vi "CASH.vi"(8 "error in (no error)":errorcluster caption="entrée d'erreur (pas d'erreur)", 11 "Portfolio en entrée":refnum<class "Portfolio.lvclass"> caption="DNL_LabVIEW Object in") -> (0 "error out":errorcluster caption="sortie d'erreur", 2 "CASH":dbl, 3 "Portfolio en sortie":refnum<class "Portfolio.lvclass"> caption="DNL_LabVIEW Object out")   [LabVIEW 2012, in "Portfolio.lvclass"]
uses:
  Portfolio.lvclass
  Portfolio.lvclass/Portfolio.ctl
  Operations/Operations.lvclass
  Exchanges/Exchanges.lvclass
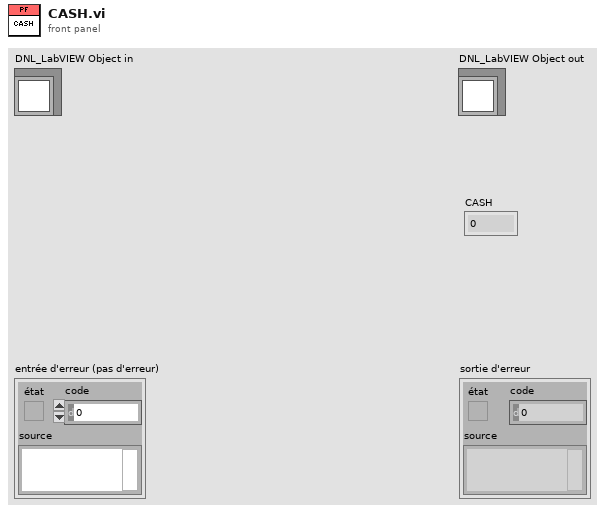
[diagram p1: front panel]
types:
  T1 = typedef "Operation Parameters.ctl" = cluster{"Date":timestamp, "Operation Type":T2, "Amount":dbl, "Comment":string, "Currency":T3}
  T2 = typedef "Operation Type Enum.ctl" = enum16{"Coupons", "Dépot", "Retrait", "Intérêts", "Taxe"}
  T3 = typedef "Currencies.ctl" = enum16{"Euro", "Dollar", "Yen", "RIM", "CHF"}
  T4 = typedef "Exchange Parameters.ctl" = cluster{"Date":timestamp, "Exchange Type":T5, "ISIN":string, "Label":string, "Price":dbl, "Qty":dbl, "Currency":T3, "Tax":dbl, "Comment":string}
  T5 = typedef "Exchange.lvclass/Exchange Type Enum.ctl" = enum16{"ACHAT", "VENTE"}
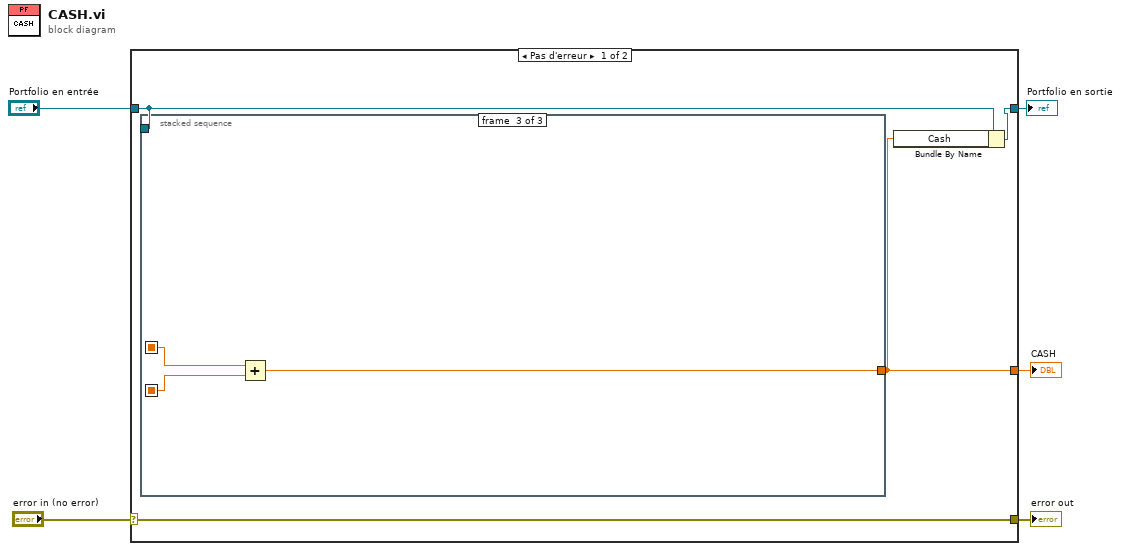
[diagram p0: block diagram]
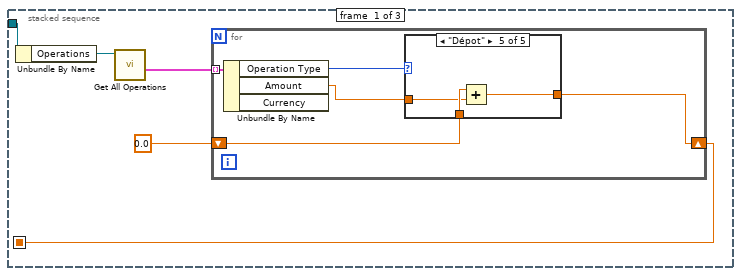
[diagram p2: hidden frame]
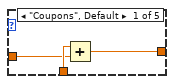
[diagram p3: hidden frame]
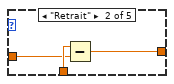
[diagram p4: hidden frame]
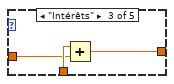
[diagram p5: hidden frame]
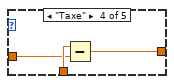
[diagram p6: hidden frame]
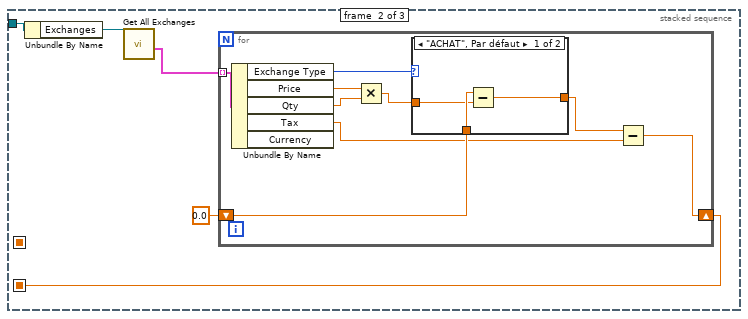
[diagram p7: hidden frame]
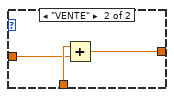
[diagram p8: hidden frame]
diagram:
  n1 = case shown="Pas d'erreur" "error in (no error)" {
    selector: "error in (no error)" -> [w9 w59]
    tunnel: [w9 w59] -> w4
    tunnel: [w7 w58] -> w2
    tunnel: "Portfolio en entrée" -> [w8 w58]
    tunnel: [w6 _] -> w1
    frame No Error {
      n2 = stacked-sequence {
        seq-local: [w10 _ _] -> [_ _ w57]
        seq-local: [_ w35 _] -> [_ _ w56]
        tunnel: w8 -> [w14 w39 _]
        tunnel: [_ _ w55] -> w6
        frame #0 {
          n3 = Unbundle By Name(w14) -> ("Operations"=w13:refnum<class "Operations.lvclass">)
          n4 = call "Get All Operations.vi"("Operations en entrée"=w13) -> ("Operations"=w12:T1[])  [unwired: 6 in, 4 out]
          n5 = for {
            tunnel: w12 -> [w19] mode=indexing
            shift-right: [w15] -> w10
            shift-left: 0.0 -> [w17]
            n6 = Unbundle By Name(w19) -> ("Operation Type"=w18:T2, "Amount"=w16:dbl)  [unwired: 1 out]
            n7 = case shown="\"Dépot\"" w18 {
              tunnel: w17 -> [w22 w25 w28 w31 w34]
              tunnel: w16 -> [w21 w24 w27 w30 w33]
              tunnel: [w20 w23 w26 w29 w32] -> w15
              frame "Coupons", Default {
                n8 = Add(x=w22, y=w21) -> (x+y=w20:dbl)
              }
              frame "Retrait" {
                n9 = Subtract(x=w25, y=w24) -> (x-y=w23:dbl)
              }
              frame "Intérêts" {
                n10 = Add(x=w28, y=w27) -> (x+y=w26:dbl)
              }
              frame "Taxe" {
                n11 = Subtract(x=w31, y=w30) -> (x-y=w29:dbl)
              }
              frame "Dépot" {
                n12 = Add(x=w34, y=w33) -> (x+y=w32:dbl)
              }
            }
          }
        }
        frame #1 {
          n13 = Unbundle By Name(w39) -> ("Exchanges"=w38:refnum<class "Exchanges.lvclass">)
          n14 = call "Get All Exchanges.vi"("Exchanges en entrée"=w38) -> ("Exchanges"=w37:T4[])  [unwired: 6 in, 4 out]
          n15 = for {
            tunnel: w37 -> [w48] mode=indexing
            shift-right: [w41] -> w35
            shift-left: 0.0 -> [w46]
            n16 = Unbundle By Name(w48) -> ("Exchange Type"=w47:T5, "Price"=w45:dbl, "Qty"=w44:dbl, "Tax"=w40:dbl)  [unwired: 1 out]
            n17 = Multiply(x=w45, y=w44) -> (x*y=w43:dbl)
            n18 = case shown="\"ACHAT\", Par défaut" w47 {
              tunnel: w46 -> [w51 w54]
              tunnel: w43 -> [w50 w53]
              tunnel: [w49 w52] -> w42
              frame "ACHAT", Default {
                n19 = Subtract(x=w51, y=w50) -> (x-y=w49:dbl)
              }
              frame "VENTE" {
                n20 = Add(x=w54, y=w53) -> (x+y=w52:dbl)
              }
            }
            n21 = Subtract(x=w42, y=w40) -> (x-y=w41:dbl)
          }
        }
        frame #2 {
          n22 = Add(x=w57, y=w56) -> (x+y=w55:dbl)
        }
      }
      n23 = Bundle By Name(cluster=w8, "Cash"=w6) -> (w7:refnum<class "Portfolio.lvclass">)
    }
    frame Error {
    }
  }
  "error out" <- w4
  "Portfolio en sortie" <- w2
  "CASH" <- w1
